vi "Initialize Time vs Numeric.vi"(8 "error in (no error)":errorcluster, 11 "Numeric Data Type in":refnum<class "Numeric Data Type.lvclass">) -> (0 "error out":errorcluster, 3 "Numeric Data Type (dup)":refnum<class "Numeric Data Type.lvclass">)   [LabVIEW 2018, in "Numeric Data Type.lvclass"]
uses:
  Numeric Data Type.lvclass
  Numeric Data Type.lvclass/Numeric Data Type.ctl
  Reference Limits Mode Tab.vi
  Reference Time-Numeric Tab.vi
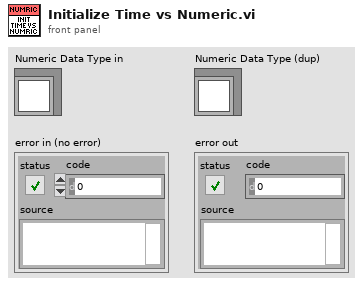
[diagram p1: front panel]
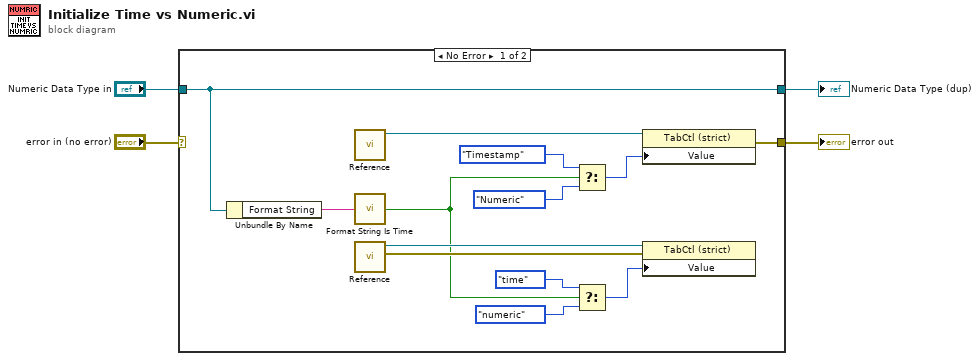
[diagram p0: block diagram]
diagram:
  n1 = case shown="No Error" "error in (no error)" {
    selector: "error in (no error)" -> [_ w18]
    tunnel: [w16 w18] -> w4
    tunnel: "Numeric Data Type in" -> [w11 w19]
    tunnel: [w11 w19] -> w1
    frame No Error {
      n2 = Unbundle By Name(w11) -> ("Format String"=w17:string)
      n3 = call-poly "Reference.vi"() -> ("Limits Mode Tab"=w12:refnum<vi>)  [unwired: 10 in, 1 out]
      n4 = call "Format String Is Time.vi"("Format String"=w17) -> ("Time?"=w8:bool)
      n5 = call-poly "Reference.vi"() -> ("error out"=w9:errorcluster, "Time/Numeric Tab"=w10:refnum<vi>)  [unwired: 10 in]
      n6 = Select(t=enum32{"Numeric", "Timestamp"}."Timestamp" ("Value"), s=w8, f=enum32{"Numeric", "Timestamp"}."Numeric" ("Value")) -> (s? t:f=w14:enum32{"Numeric", "Timestamp"})
      n7 = Select(t=enum32{"numeric", "time"}."time" ("Desired Tab"), s=w8, f=enum32{"numeric", "time"}."numeric" ("Desired Tab")) -> (s? t:f=w6:enum32{"numeric", "time"})
      n8 = property class="TabCtl (strict)"(reference=w12, "Value"=w14) -> (error out=w16:errorcluster)  [unwired: 1 in, 1 out]
      n9 = property class="TabCtl (strict)"(reference=w10, error in=w9, "Value"=w6) -> ()  [unwired: 2 out]
    }
    frame Error {
    }
  }
  "error out" <- w4
  "Numeric Data Type (dup)" <- w1
